vi "Send TCP Data (1D).vi"(0 "connection ID":refnum<k5>, 1 "Data in":dbl[](array[numeric]), 3 "error in (no error)":errorcluster, 4 "Single precision?":bool=TRUE) -> (7 "connection ID 2":refnum<k5>, 10 "error out":errorcluster)   [LabVIEW 2015]
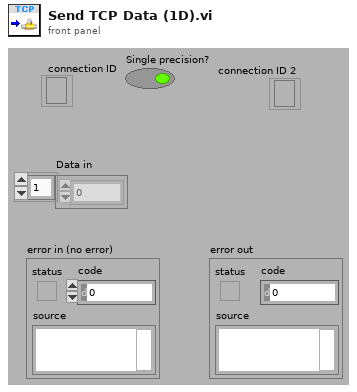
[diagram p1: front panel]
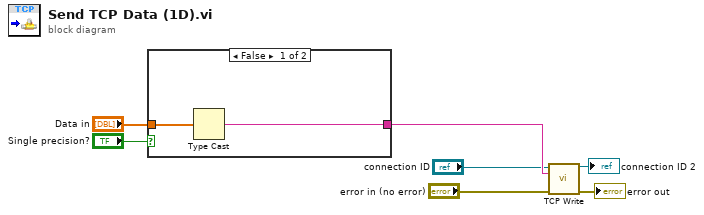
[diagram p0: block diagram]
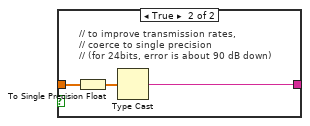
[diagram p2: hidden frame]
diagram:
  n1 = case shown="False" "Single precision?" {
    tunnel: [w9 w11] -> w6
    tunnel: "Data in" -> [w8 w10]
    frame False {
      n2 = Type Cast(x=w8) -> (*(type *) &x=w9:string)  [unwired: 1 in]
    }
    frame True {
      # "// to improve transmission rates,\n// coerce to single precision\n// (for 24bits, error is about 90 dB down)"
      n3 = To Single Precision Float(number=w10) -> (single precision float=w12:sgl[])
      n4 = Type Cast(x=w12) -> (*(type *) &x=w11:string)  [unwired: 1 in]
    }
  }
  n5 = call "TCP Write.vi"("connection ID"="connection ID", "data string"=w6, "error in (no error)"="error in (no error)") -> ("connection ID out"=→"connection ID 2":refnum<k5>, "error out"=→"error out":errorcluster)  [unwired: 10 in, 1 out]
